vi "Create Image Saving Folder.vi"(0 "Camera Prime95B Controller in":refnum<class "CameraController.lvclass">, 5 "Save Path":path, 7 "File suffix":string, 9 "StreamToDisk?":bool, 11 "error in (no error)":errorcluster, 12 "SnapShot?":bool) -> (4 "Camera Prime95B Controller out":refnum<class "CameraController.lvclass">, 6 "Saving Path":path, 8 "Stream Saving Path":path, 10 "Snap Shot Path":path, 15 "error out":errorcluster)   [LabVIEW 2020, in "CameraController.lvlib" / "CameraController.lvclass"]
uses:
  CameraController.lvclass
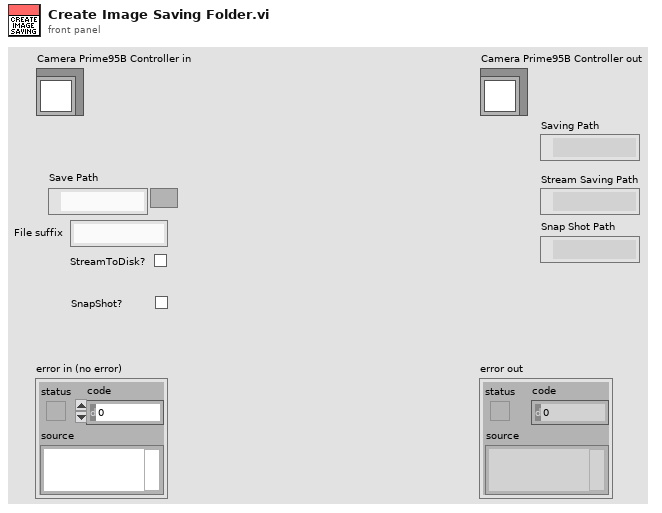
[diagram p1: front panel]
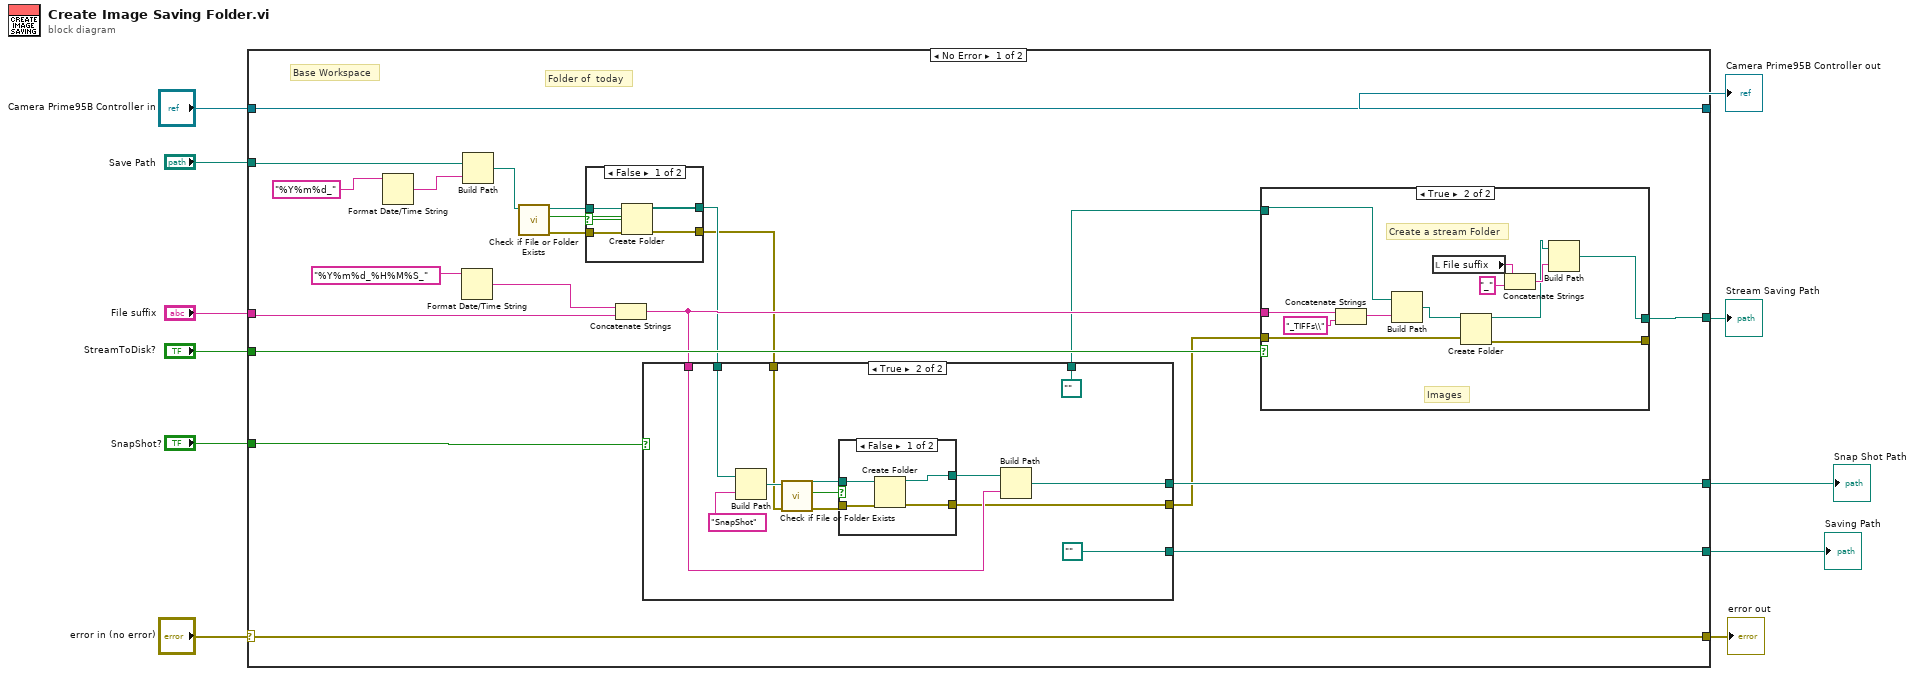
[diagram p0: block diagram]
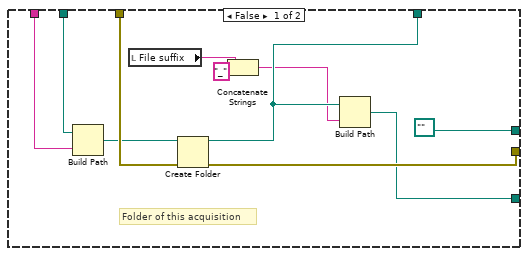
[diagram p2: hidden frame]
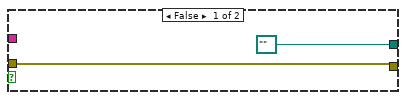
[diagram p4: hidden frame]
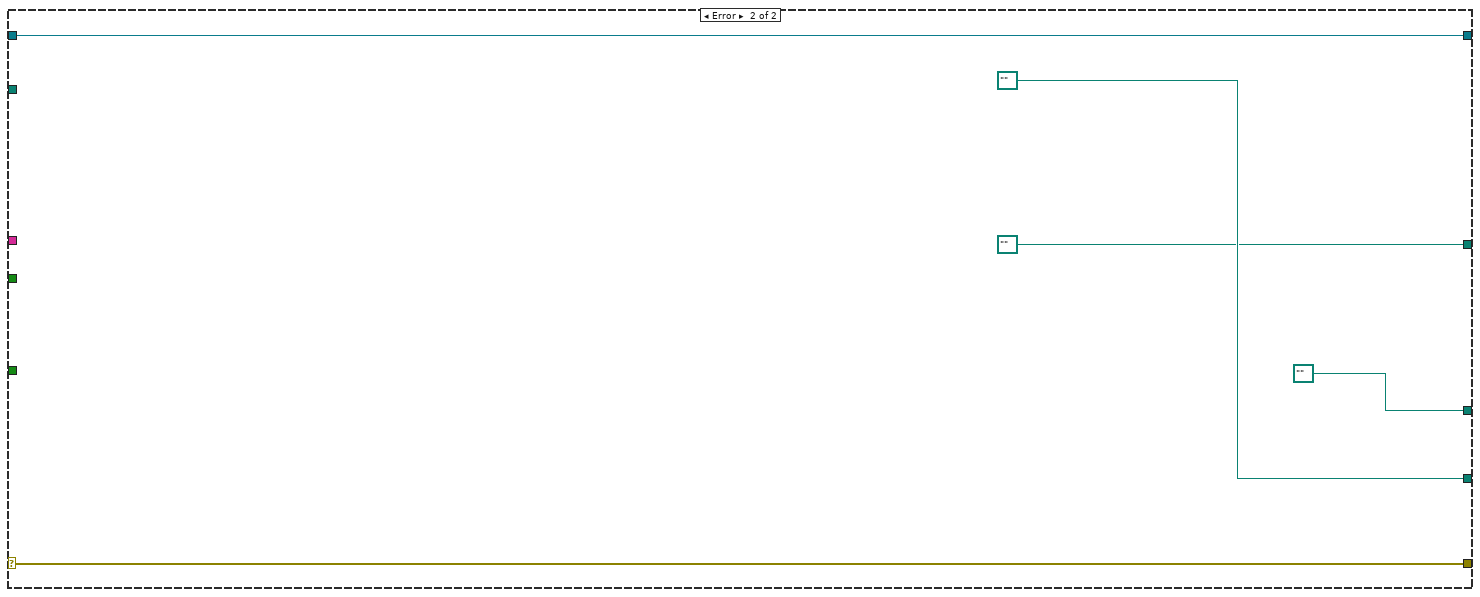
[diagram p6: hidden frame]
diagram:
  n1 = case shown="No Error" "error in (no error)" {
    selector: "error in (no error)" -> [w32 w88]
    tunnel: [w32 w88] -> w10
    tunnel: [w33 w87] -> w8
    tunnel: "Camera Prime95B Controller in" -> [w33 w87]
    tunnel: "Save Path" -> [w23 _]
    tunnel: "File suffix" -> [w22 _]
    tunnel: "StreamToDisk?" -> [w21 _]
    tunnel: [w20 path "" ("created path")] -> w3
    tunnel: [w12 path "" ("created path")] -> w4
    tunnel: "SnapShot?" -> [w19 _]
    tunnel: [w18 path "" ("appended path")] -> w1
    frame No Error {
      # "Base Workspace"
      # "Folder of  today"
      n2 = Format Date/Time String(time format string (%c)="%Y%m%d_") -> (date/time string=w26:string)  [unwired: 2 in]
      n3 = Format Date/Time String(time format string (%c)="%Y%m%d_%H%M%S_") -> (date/time string=w31:string)  [unwired: 2 in]
      n4 = Build Path(base path=w23, name or relative path=w26) -> (appended path=w27:path)
      n5 = call <vilib>:"Check if File or Folder Exists.vi"("path"=w27) -> ("error out"=w30:errorcluster, "file or folder exists?"=w28:bool, "dup path"=w29:path)  [unwired: 8 in]
      n6 = case shown="False" w28 {
        tunnel: w29 -> [w81 w83]
        tunnel: [w80 w82] -> w15
        tunnel: [w79 w83] -> w16
        tunnel: w30 -> [w78 w82]
        frame False {
          n7 = Create Folder(path (use dialog)=w81, error in=w78) -> (created path=w79:path, error out=w80:errorcluster)  [unwired: 1 in, 1 out]
        }
        frame True {
        }
      }
      n8 = Concatenate Strings(w31, w22) -> (w17:string)
      n9 = case shown="True" w19 {
        tunnel: w16 -> [w38 w57]
        tunnel: [path "" ("appended path") w50] -> w18
        tunnel: w17 -> [w43 w49]
        tunnel: w15 -> [w42 w48]
        tunnel: [w40 w47] -> w14
        tunnel: [w39 path "" ("created path")] -> w13
        tunnel: [w34 path "" ("appended path")] -> w12
        frame False {
          # "Folder of this acquisition"
          n10 = Build Path(base path=w38, name or relative path=w43) -> (appended path=w41:path)
          n11 = local read "File suffix"() -> (w36:string)
          n12 = Create Folder(path (use dialog)=w41, error in=w42) -> (created path=w39:path, error out=w40:errorcluster)  [unwired: 1 in, 1 out]
          n13 = Concatenate Strings(w36, "_" ("string")) -> (w37:string)
          n14 = Build Path(base path=w39, name or relative path=w37) -> (appended path=w34:path)
        }
        frame True {
          n15 = Build Path(base path=w57, name or relative path="SnapShot") -> (appended path=w55:path)
          n16 = call <vilib>:"Check if File or Folder Exists.vi"("error in (no error)"=w48, "path"=w55) -> ("error out"=w52:errorcluster, "file or folder exists?"=w54:bool, "dup path"=w53:path)  [unwired: 7 in]
          n17 = case shown="False" w54 {
            tunnel: w53 -> [w61 w63]
            tunnel: [w60 w62] -> w47
            tunnel: [w59 w63] -> w51
            tunnel: w52 -> [w58 w62]
            frame False {
              n18 = Create Folder(path (use dialog)=w61, error in=w58) -> (created path=w59:path, error out=w60:errorcluster)  [unwired: 1 in, 1 out]
            }
            frame True {
            }
          }
          n19 = Build Path(base path=w51, name or relative path=w49) -> (appended path=w50:path)
        }
      }
      n20 = case shown="True" w21 {
        tunnel: [path "" ("created path") w66] -> w20
        tunnel: w14 -> [w65 w77]
        tunnel: [w65 w76] -> _
        tunnel: w13 -> [_ w75]
        tunnel: w17 -> [_ w73]
        frame False {
        }
        frame True {
          # "Create a stream Folder"
          # "Images"
          n21 = Concatenate Strings(w73, "_TIFFs\\" ("string")) -> (w71:string)
          n22 = Build Path(base path=w75, name or relative path=w71) -> (appended path=w74:path)
          n23 = local read "File suffix"() -> (w68:string)
          n24 = Create Folder(path (use dialog)=w74, error in=w77) -> (created path=w67:path, error out=w76:errorcluster)  [unwired: 1 in, 1 out]
          n25 = Concatenate Strings(w68, "_" ("string")) -> (w69:string)
          n26 = Build Path(base path=w67, name or relative path=w69) -> (appended path=w66:path)
        }
      }
    }
    frame Error {
    }
  }
  "error out" <- w10
  "Camera Prime95B Controller out" <- w8
  "Saving Path" <- w4
  "Stream Saving Path" <- w3
  "Snap Shot Path" <- w1
